vi "GV gated pixel clock change.vi"() -> ()   [LabVIEW 2017]
panel:
  out "Gated pixel clock change":bool
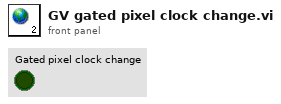
[diagram p1: front panel]
diagram:
